vi "DAC Configure.vi"(8 "error in":errorcluster, 11 "DAC Heater Box Temperatures in":refnum<class "DAC Heater Box Temperatures.lvclass">) -> (0 "error out":errorcluster, 3 "DAC Heater Box Temperatures out":refnum<class "DAC Heater Box Temperatures.lvclass">)   [LabVIEW 2019, in "DAC.lvlib" / "DAC Heater Box Temperatures.lvclass"]
uses:
  DAC Heater Box Temperatures.lvclass
  C:/Users/wg/Documents/LV_Projects/TestStand/App/DAC/DAC.lvclass
  DAC.lvclass/DAC.ctl
  DAC Heater Box Temperatures.lvclass/DAC Heater Box Temperatures.ctl
  <vilib>/DAQmx/create/channels.llb/DAQmx Create Channel (AI-Temperature-RTD).vi
  DAC.lvclass
  <resource>/objmgr/daqmx.rc
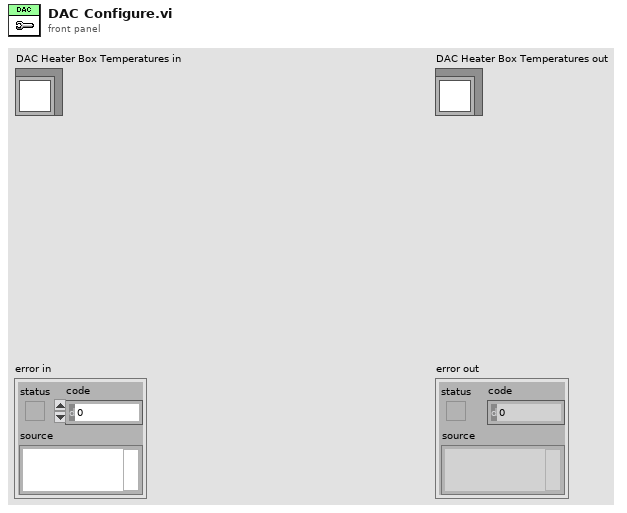
[diagram p1: front panel]
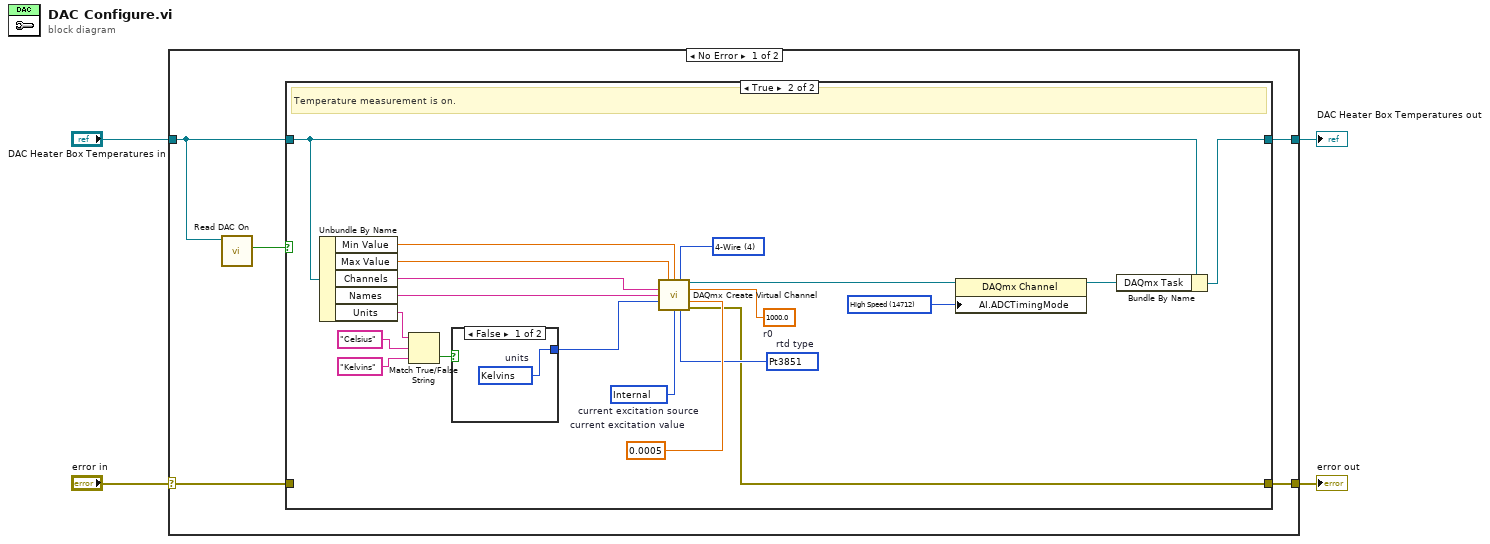
[diagram p0: block diagram]
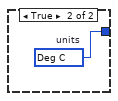
[diagram p3: hidden frame]
diagram:
  n1 = case shown="No Error" "error in" {
    selector: "error in" -> [w6 w35]
    tunnel: [w5 w35] -> w4
    tunnel: [w7 w34] -> w3
    tunnel: "DAC Heater Box Temperatures in" -> [w9 w34]
    frame No Error {
      n2 = call "Read DAC On.vi"("DAC in"=w9) -> ("DAC On"=w8:bool)  [unwired: 8 in, 2 out]
      n3 = case shown="True" w8 {
        tunnel: w9 -> [w11 w20]
        tunnel: [w11 w19] -> w7
        tunnel: w6 -> [w10 _]
        tunnel: [w10 w18] -> w5
        frame False {
          # "Temperature measurement is off."
        }
        frame True {
          w12 = 14712 items=["Automatic"=16097, "High Resolution"=10195, "High Speed"=14712, "Best 50 Hz Rejection"=14713, "Best 60 Hz Rejection"=14714, "Custom"=10137] ("AI.ADCTimingMode")
          w29 = 0.0005  # current excitation value
          w28 = 10200 items=["Internal"=10200, "External"=10167, "None"=10230]  # current excitation source
          w30 = 1000.0  # r0
          w31 = 4 items=["2-Wire"=2, "3-Wire"=3, "4-Wire"=4] ("resistance configuration")
          w27 = 10071 items=["Pt3750"=12481, "Pt3851"=10071, "Pt3911"=12482, "Pt3916"=10069, "Pt3920"=10053, "Pt3928"=12483, "Custom"=10137]  # rtd type
          # "Temperature measurement is on."
          n4 = Unbundle By Name(w20) -> ("Min Value"=w21:dbl, "Max Value"=w22:dbl, "Channels"=w17:string, "Names"=w15:string, "Units"=w16:string)
          n5 = Match True/False String(2:"Kelvins" ("false string"), 3:"Celsius" ("true string"), 4:w16) -> (0:w24:bool)  [unwired: 1 out]
          n6 = case shown="False" w24 {
            tunnel: [w32 w33] -> w23
            frame False {
              w32 = 10325 items=["Deg C"=10143, "Deg F"=10144, "Kelvins"=10325, "Deg R"=10145, "From Custom Scale"=10065]  # units
            }
            frame True {
              w33 = 10143 items=["Deg C"=10143, "Deg F"=10144, "Kelvins"=10325, "Deg R"=10145, "From Custom Scale"=10065]  # units
            }
          }
          n7 = call-poly <vilib>:"DAQmx Create Virtual Channel.vi"("maximum value"=w22, "minimum value"=w21, "resistance configuration"=w31, "physical channels"=w17, "r0"=w30, "name to assign"=w15, "units"=w23, "current excitation value"=w29, "current excitation source"=w28, "rtd type"=w27) -> ("task out"=w14:refnum<k21>, "error out"=w18:errorcluster)  [unwired: 4 in]
          n8 = property class="DAQmx Channel"(reference=w14, "AI.ADCTimingMode"=w12) -> (reference out=w13:refnum<k21>)  [unwired: 1 in, 1 out]
          n9 = Bundle By Name(cluster=w20, "DAQmx Task"=w13) -> (w19:refnum<class "DAC Heater Box Temperatures.lvclass">)
        }
      }
    }
    frame Error {
    }
  }
  "error out" <- w4
  "DAC Heater Box Temperatures out" <- w3
